vi "CheesyDrive.vi"(6 "Quickturn":bool, 8 "QuickTurn Sensitivty":dbl=0.7, 9 "Sensitivty":dbl=1.0, 10 "Wheel":dbl(slide) scale=-1.0..1.0, 11 "Throttle":dbl(slide)=0.007874015748031496 scale=-1.0..1.0) -> (2 "Right PWM":dbl, 3 "Left PWM":dbl)   [LabVIEW 2016]
panel:
  in  "alpha":dbl=0.1
  out "Waveform Chart":dbl(graph)
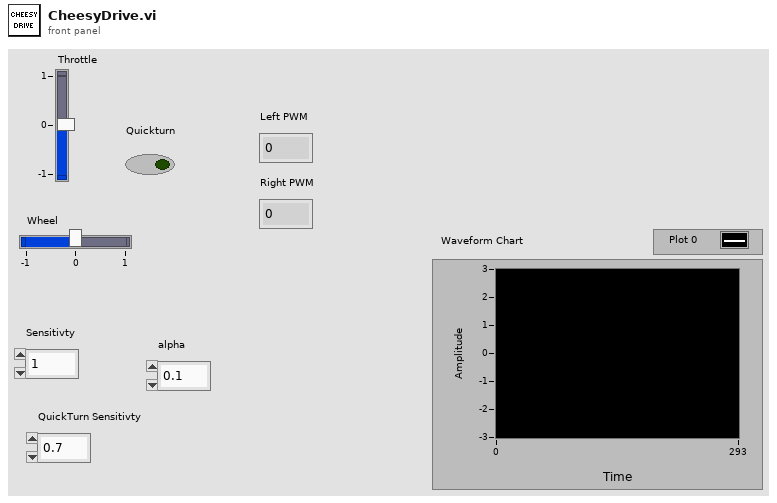
[diagram p1: front panel]
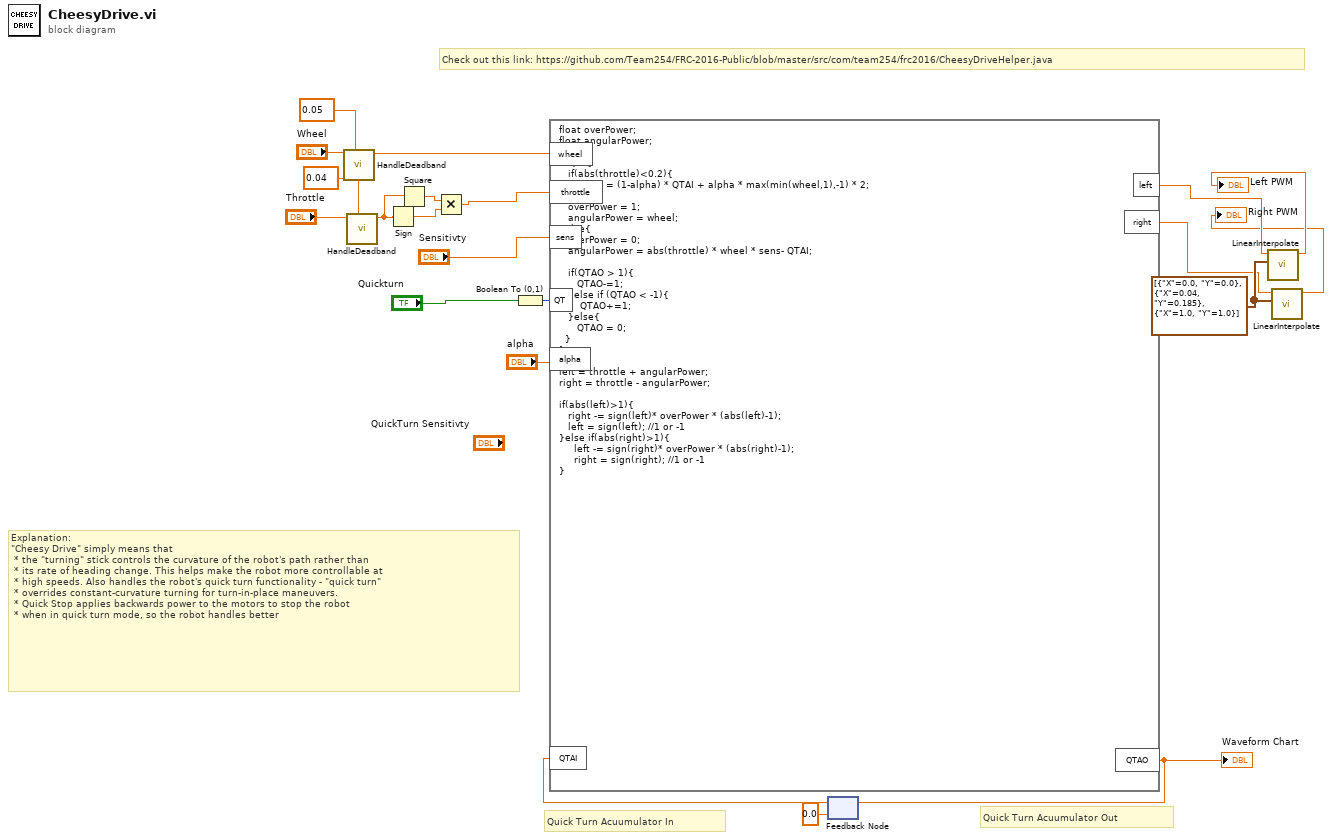
[diagram p0: block diagram]
diagram:
  w5 = cluster{"X":dbl, "Y":dbl}[] [{"X"=0.0, "Y"=0.0}, {"X"=0.04, "Y"=0.185}, {"X"=1.0, "Y"=1.0}] ("Points")
  # "Explanation:\n\"Cheesy Drive\" simply means that\n * the \"turning\" stick controls the curvature of the robot's path rather than\n * its rate of heading change. This helps make the robot more controllable at\n * high speeds. Also handles the robot's quick turn functionality - \"quick turn\"\n * overrides constant-curvature turning for turn-in-place maneuvers.\n * Quick Stop applies backwards power to the motors to stop the robot\n * when in quick turn mode, so the robot handles better"
  # "Quick Turn Acuumulator Out"
  # "Quick Turn Acuumulator In"
  # "Check out this link: https://github.com/Team254/FRC-2016-Public/blob/master/src/com/team254/frc2016/CheesyDriveHelper.java"
  n1 = call "HandleDeadband.vi"("Deadband"=0.05, "Input"="Wheel") -> ("Output"=w18:dbl)  [unwired: 9 in]
  n2 = call "HandleDeadband.vi"("Deadband"=0.04, "Input"="Throttle") -> ("Output"=w8:dbl)  [unwired: 9 in]
  n3 = Sign(1:w8) -> (0:w7:dbl)
  n4 = Square(x=w8) -> (x^2=w9:dbl)
  n5 = Multiply(x=w9, y=w7) -> (x*y=w6:dbl)
  n6 = Boolean To (0,1)(Boolean="Quickturn") -> (0, 1=w13:i16)
  n7 = feedback #1(0.0 ("QTAccumulatorO")) -> (w11:dbl)
  n8 = formula code="float overPower;\nfloat angularPower;\n\nif(QT){\n   if(abs(throttle)<0.2){\n      QTAO = (1-alpha) * QTAI + alpha * max(min(wheel,1),-1) * 2;\n   }\n   overPower = 1;\n   angularPower = wheel;\n}else{\n   overPower = 0;\n   angularPower = abs(throttle) * wheel * sens- QTAI;\n\n   if(QTAO > 1){\n      QTAO-=1;\n   }else if (QTAO < -1){\n       QTAO+=1;\n   }else{\n      QTAO = 0;\n  }\n}\n\nleft = throttle + angularPower;\nright = throttle - angularPower;\n\nif(abs(left)>1){\n   right -= sign(left)* overPower * (abs(left)-1);\n   left = sign(left); //1 or -1\n}else if(abs(right)>1){\n     left -= sign(right)* overPower * (abs(right)-1);\n     right = sign(right); //1 or -1 \n}"("wheel"=w18, "throttle"=w6, "sens"="Sensitivty", "QT"=w13, "alpha"="alpha", "QTAI"=w11) -> ("left"=w3:dbl, "right"=w4:dbl, "QTAO"=w14:dbl)
  "Waveform Chart" <- w14
  n9 = feedback-in #1(w14) -> ()
  n10 = call "LinearInterpolate.vi"("Points"=w5, "Value"=w3) -> ("Output"=→"Left PWM":dbl)  [unwired: 9 in]
  n11 = call "LinearInterpolate.vi"("Points"=w5, "Value"=w4) -> ("Output"=→"Right PWM":dbl)  [unwired: 9 in]
